vi "Help--Const.vi"() -> (3 "Help Command":string)   [LabVIEW 2017, in "Communications Library.lvlib"]
uses:
  Communications Library.lvlib
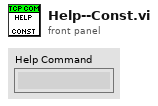
[diagram p1: front panel]
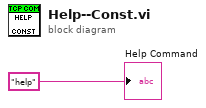
[diagram p0: block diagram]
diagram:
  "Help Command" <- "help" ("data in")
